vi "FindHome_MultiAxis.vi"(0 "Bd ID In":T3=1, 5 "Axis":T1=1 items=["Axis 1"=1, "Axis 2"=2, "Axis 3"=3, "Axis 4"=4, "Axis 5"=5, "Axis 6"=6, "Axis 7"=7, "Axis 8"=8], 11 "error in":errorcluster, 12 "Velocity (Degrees/s)":dbl=6.0 caption="Degrees/s", 13 "Accel/Decel (Degrees/s/s)":dbl=3.0 caption="Degrees/s^2" format="%.2f") -> (4 "Bd ID Out":T3, 6 "Axis Resource Output":T2 items=["Axis Control"=0, "Axis 1"=1, "Axis 2"=2, "Axis 3"=3, "Axis 4"=4, "Axis 5"=5, "Axis 6"=6, "Axis 7"=7, "Axis 8"=8, "Vector Space Control"=16, "Vector Space 1"=17, "Vector Space 2"=18, "Vector Space 3"=19, "Vector Space 4"=20, "Encoder Control"=32, "Encoder 1"=33, "Encoder 2"=34, "Encoder 3"=35, "Encoder 4"=36, "Encoder 5"=37, "Encoder 6"=38, "Encoder 7"=39, "Encoder 8"=40, "DAC Channel 1"=49, "DAC Channel 2"=50, "DAC Channel 3"=51, "DAC Channel 4"=52, "DAC Channel 5"=53, "DAC Channel 6"=54, "DAC Channel 7"=55, "DAC Channel 8"=56, "Stepper Output 1"=65, "Stepper Output 2"=66, "Stepper Output 3"=67, "Stepper Output 4"=68, "Stepper Output 5"=69, "Stepper Output 6"=70, "Stepper Output 7"=71, "Stepper Output 8"=72, "ADC Channel 1"=81, "ADC Channel 2"=82, "ADC Channel 3"=83, "ADC Channel 4"=84, "ADC Channel 5"=85, "ADC Channel 6"=86, "ADC Channel 7"=87, "ADC Channel 8"=88], 15 "error out":errorcluster)   [LabVIEW 2010]
doc: "Finds the reference home position for a given axis of the PUMA 560 and resets encoder counts to zero when found. \n\nNotes: \nHome position is determined by values of the absolute position potentiometer voltage corresponding to the PUMA 560's engraved home position markers.\n\nFunction is configured as re-entrant type to allow multiple instances of the VI to execute in parallel.\n\nSometimes an axis will not stop at its home position. This is a tuning problem; if the axis is tuned poorly it is unable to stop exactly at the home position."
uses:
  <vilib>/Motion/FlexMotion/CustomControls/CustomControls.llb/Resource Out (Enum).flx
  <vilib>/Motion/FlexMotion/CustomControls/CustomControls.llb/Axis To Control.flx
  Typedefs/Units_Enum.ctl
  Globals/AxisSpace.vi
  <vilib>/Motion/FlexMotion/FunctionsVIs/StartStopMotion.llb/Start Motion (8 axes).flx
  <vilib>/Motion/FlexMotion/FunctionsVIs/StartStopMotion.llb/Stop Motion (8 axes).flx
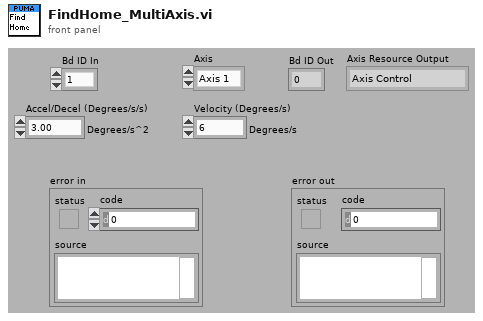
[diagram p1: front panel]
types:
  T1 = typedef "Axis To Control.flx" = u16
  T2 = typedef "Resource Out (Enum).flx" = u16
  T3 = typedef "Bd Id Out" = u8
  T4 = typedef "AxisSpaceCfg_ArrayofAxisCfg.ctl" = T5[]
  T5 = typedef "AxisCfg_cluster.ctl" = cluster{"Axis":T6, "Counts/Rev":dbl, "Gear Ratio":dbl, "Home Position":dbl}
  T6 = typedef "Axis To Read.flx" = u16
  T7 = typedef "Units_Enum.ctl" = enum16{"Radians", "Encoder Counts", "Revolutions", "Degrees"}
  T8 = enum16{"Absolute Position", "Relative Position", "Velocity", "Relative to Cap Pos", "Modulus Position", "Absolute Contouring", "Relative Contouring"}
  T9 = cluster{"Run/Stop":bool, "Profile Complete":bool, "Motor Off ":bool, "Following Error":bool, "Limit Switch":bool, "Home Switch":bool, "SW Limit Switch":bool, "Watchdog":bool, "Velocity Threshold":bool, "Position Brkpt":bool, "Home Found":bool, "Index Found":bool, "High Speed Capture":bool, "Reverse Direction":bool, "Blend Complete":bool, "Move Complete":bool}
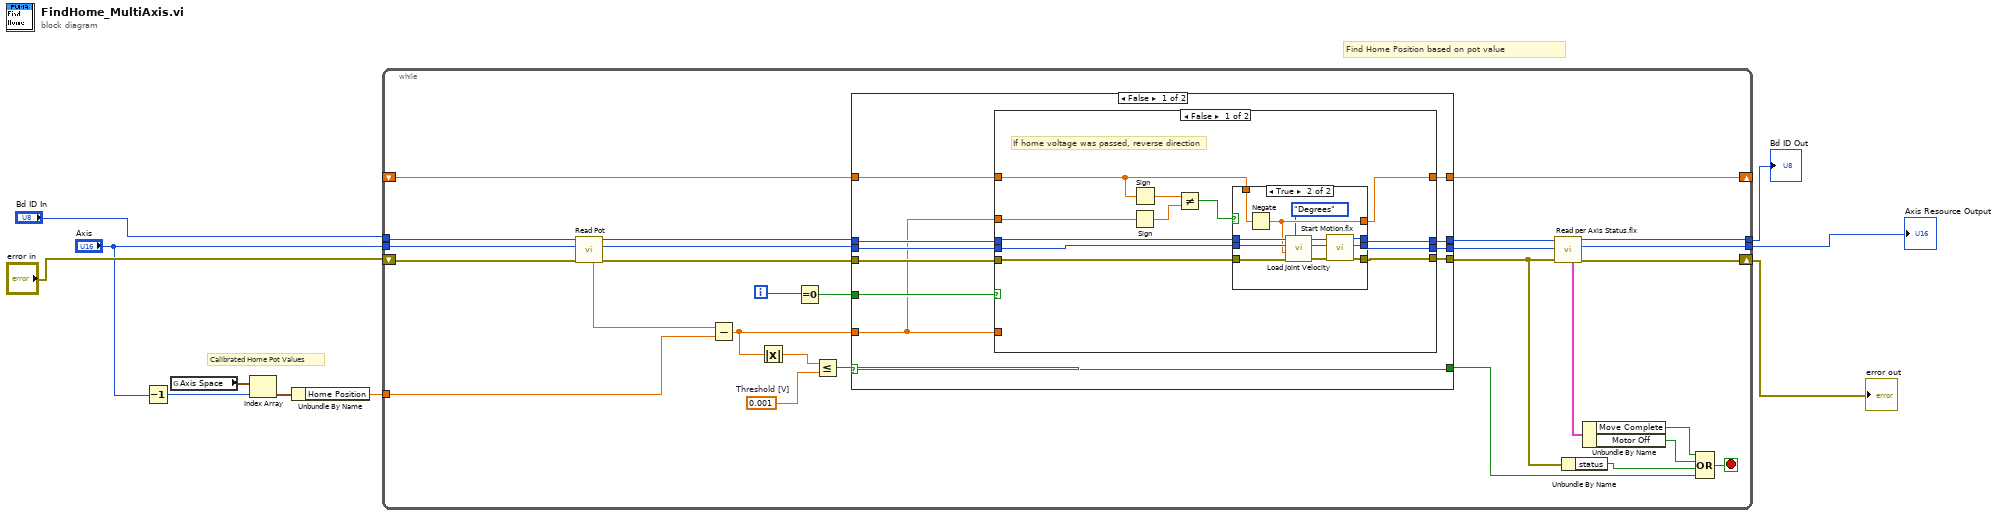
[diagram p0: block diagram]
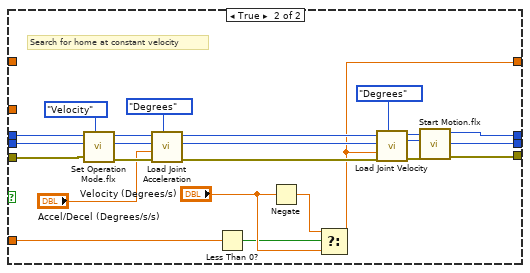
[diagram p3: hidden frame]
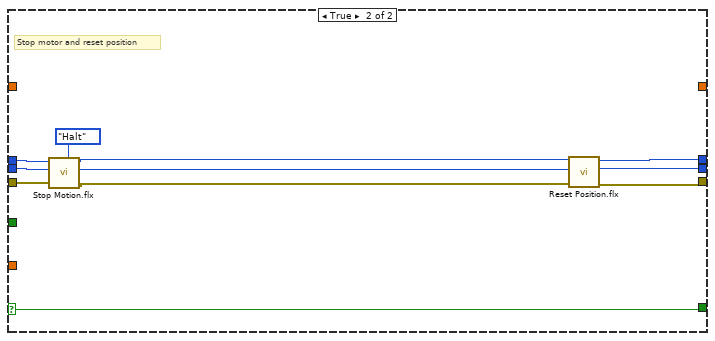
[diagram p4: hidden frame]
diagram:
  # "Calibrated Home Pot Values"
  # "Find Home Position based on pot value"
  n1 = Decrement(x="Axis") -> (x-1=w4:T1)
  n2 = global read "AxisSpace.vi" "Axis Space"() -> (w3:T4)
  n3 = Index Array(array=w3, index=w4) -> (element=w5:T5)
  n4 = Unbundle By Name(w5) -> ("Home Position"=w1:dbl)
  n5 = while {
    tunnel: "Bd ID In" -> [w30]
    tunnel: [w20] -> w8
    tunnel: [w19] -> w7
    shift-right: [w22] -> w6
    shift-left: "error in" -> [w27]
    tunnel: "Axis" -> [w14]
    shift-right: [w13] -> _
    shift-left: _ -> [w12]
    tunnel: w1 -> [w11]
    i -> [w36]
    stop <- w35 stop-if-true
    w38 = 0.001  # Threshold [V]
    n6 = call "Read Pot.vi"("error in (no error)"=w27, "Axis In"=w14, "Board ID"=w30) -> ("error out"=w26:errorcluster, "Axis Out"=w28:T1, "Bd ID Out"=w29:T3, "Pot Voltage"=w16:dbl)  [unwired: 5 in]
    n7 = Subtract(x=w16, y=w11) -> (x-y=w25:dbl)
    n8 = Absolute Value(x=w25) -> (abs(x)=w34:dbl)
    n9 = Equal To 0?(x=w36) -> (x = 0?=w31:bool)
    n10 = Less Or Equal?(x=w34, y=w38) -> (x <= y?=w37:bool)
    n11 = case shown="False" w37 {
      selector: w37 -> [w49 w112]
      tunnel: [w49 w112] -> w32
      tunnel: [w48 w110] -> w24
      tunnel: [w47 w109] -> w23
      tunnel: [w46 w108] -> w21
      tunnel: w29 -> [w44 w107]
      tunnel: w31 -> [w45 _]
      tunnel: w25 -> [w39 _]
      tunnel: w28 -> [w43 w103]
      tunnel: w26 -> [w42 w102]
      tunnel: [w41 _] -> w13
      tunnel: w12 -> [w40 _]
      frame False {
        n12 = case shown="False" w45 {
          tunnel: [w52 w101] -> w48
          tunnel: [w51 w100] -> w47
          tunnel: [w58 w99] -> w46
          tunnel: w44 -> [w55 w91]
          tunnel: w43 -> [w56 w86]
          tunnel: w42 -> [w57 w85]
          tunnel: [w53 w80] -> w41
          tunnel: w40 -> [w54 _]
          tunnel: w39 -> [w50 _]
          tunnel: w39 -> [_ w79]
          frame False {
            # "If home voltage was passed, reverse direction"
            n13 = Sign(1:w50) -> (0:w61:dbl)
            n14 = Sign(1:w54) -> (0:w59:dbl)
            n15 = Not Equal?(x=w59, y=w61) -> (x != y?=w60:bool)
            n16 = case shown="True" w60 {
              tunnel: [w63 w71] -> w58
              tunnel: w57 -> [w63 w77]
              tunnel: w55 -> [w65 w75]
              tunnel: w56 -> [w64 w76]
              tunnel: [w65 w67] -> w52
              tunnel: [w64 w70] -> w51
              tunnel: w54 -> [w62 w74]
              tunnel: [w62 w73] -> w53
              frame False {
              }
              frame True {
                n17 = Negate(x=w74) -> (-x=w73:dbl)
                n18 = call "Load Joint Velocity.vi"("Units (Encoder Counts)"=Units_Enum."Degrees", "error in (no error)"=w77, "Velocity"=w73, "Axis"=w76, "Board ID"=w75) -> ("error out"=w72:errorcluster, "Resource Output"=w69:T2, "Bd ID Out"=w68:T3)  [unwired: 4 in]
                n19 = call-poly <vilib>:"Start Motion.flx"("error in (no error)"=w72, "Axis or Vector Space"=w69, "Board ID"=w68) -> ("error out"=w71:errorcluster, "Resource Output"=w70:T2, "Bd ID Out"=w67:T3)  [unwired: 3 in]
              }
            }
          }
          frame True {
            # "Search for home at constant velocity"
            n20 = call <vilib>:"Set Operation Mode.flx"("Position Mode (Absolute)"=T8."Velocity", "error in (no error)"=w85, "Axis or Vector Space"=w86, "Board ID"=w91) -> ("error out"=w88:errorcluster, "Resource Output"=w89:T2, "Bd ID Out"=w90:T3)  [unwired: 2 in]
            n21 = call "Load Joint Acceleration.vi"("Units (Encoder Counts)"=Units_Enum."Degrees", "error in (no error)"=w88, "Acceleration"="Accel/Decel (Degrees/s/s)", "Axis"=w89, "Board ID"=w90) -> ("error out"=w92:errorcluster, "Resource Output"=w93:T2, "Bd ID Out"=w94:T3)  [unwired: 4 in]
            n22 = Less Than 0?(x=w79) -> (x < 0?=w78:bool)
            n23 = Negate(x="Velocity (Degrees/s)") -> (-x=w82:dbl)
            n24 = Select(t=w82, s=w78, f="Velocity (Degrees/s)") -> (s? t:f=w80:dbl)
            n25 = call "Load Joint Velocity.vi"("Units (Encoder Counts)"=Units_Enum."Degrees", "error in (no error)"=w92, "Velocity"=w80, "Axis"=w93, "Board ID"=w94) -> ("error out"=w97:errorcluster, "Resource Output"=w96:T2, "Bd ID Out"=w95:T3)  [unwired: 4 in]
            n26 = call-poly <vilib>:"Start Motion.flx"("error in (no error)"=w97, "Axis or Vector Space"=w96, "Board ID"=w95) -> ("error out"=w99:errorcluster, "Resource Output"=w100:T2, "Bd ID Out"=w101:T3)  [unwired: 3 in]
          }
        }
      }
      frame True {
        # "Stop motor and reset position"
        n27 = call-poly <vilib>:"Stop Motion.flx"("Stop Type (Decel)"=enum16{"Decelerate", "Halt", "Kill"}."Halt", "error in (no error)"=w102, "Axis or Vector Space"=w103, "Board ID"=w107) -> ("error out"=w104:errorcluster, "Resource Output"=w105:T2, "Bd ID Out"=w106:T3)  [unwired: 3 in]
        n28 = call <vilib>:"Reset Position.flx"("error in (no error)"=w104, "Axis"=w105, "Board ID"=w106) -> ("error out"=w108:errorcluster, "Resource Output"=w109:T2, "Bd ID Out"=w110:T3)  [unwired: 4 in]
      }
    }
    n29 = call <vilib>:"Read per Axis Status.flx"("error in (no error)"=w21, "Axis"=w23, "Board ID"=w24) -> ("error out"=w22:errorcluster, "Resource Output"=w19:T2, "Bd ID Out"=w20:T3, "Per Axis H/W Status"=w18:T9)  [unwired: 3 in]
    n30 = Unbundle By Name(w21) -> ("status"=w33:bool)
    n31 = Unbundle By Name(w18) -> ("Move Complete"=w15:bool, "Motor Off"=w17:bool)
    n32 = Compound Arithmetic op=OR(w15, w17, w33, w32) -> (w35:bool)
  }
  "Bd ID Out" <- w8
  "error out" <- w6
  "Axis Resource Output" <- w7
